vi "Fetch Class Documentation.vi"(8 "error in":errorcluster {"code" format="Error %.0f"}, 10 "Parser Settings":T1, 11 "Class in":refnum<vi>) -> (0 "error out":errorcluster {"code" format="Error %.0f"}, 3 "Class Documentation Out":refnum<class "Class Documentation.lvclass">)   [LabVIEW 2023, in "VIDoc Parsing.lvlib" / "Class Documentation.lvclass"]
doc: "Takes a Class Reference in and parses out all Class Documentation information needed for document generation."
uses:
  Class Documentation.lvclass
  Settings/Parser Settings/Parser Settings Cluster.ctl
  Settings/Parser Settings/Draw Controls Cluster.ctl
  Settings/Parser Settings/Draw Option Enum.ctl
  Class Documentation.lvclass/Class Documentation.ctl
  c4881257-149c-4e35-87db-cabb12afb1ac.vi
  VIDoc Parsing.lvlib
  Settings/Parser Settings/Parser Settings.lvclass
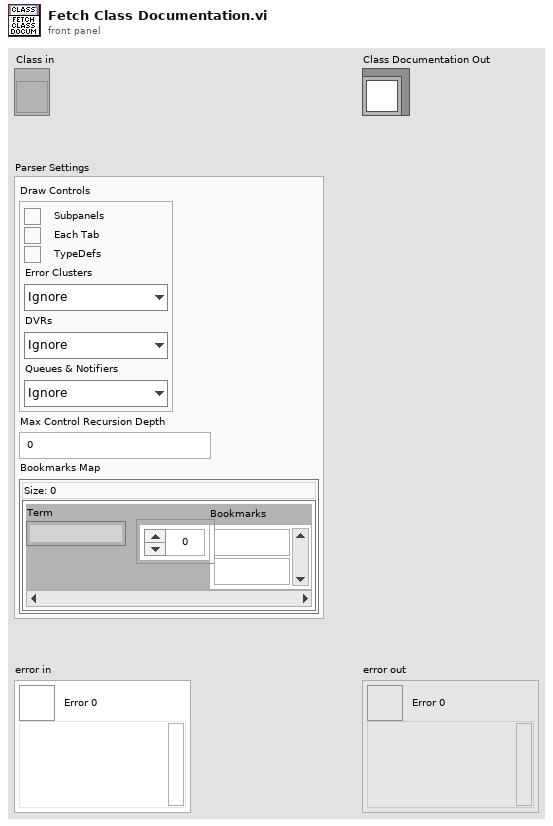
[diagram p1: front panel]
types:
  T1 = typedef "VIDoc Parsing.lvlib/Parser Settings.lvclass/Parser Settings Cluster.ctl" = cluster{"Draw Controls":T2, "Max Control Recursion Depth":i32, "Bookmarks Map":map{string, string[]}}
  T2 = typedef "VIDoc Parsing.lvlib/Parser Settings.lvclass/Draw Controls Cluster.ctl" = cluster{"Subpanels":bool, "Tabs":bool, "TypeDefs":bool, "Error Clusters":T3, "DVRs":T3, "Queues & Notifiers":T3}
  T3 = typedef "VIDoc Parsing.lvlib/Parser Settings.lvclass/Draw Option Enum.ctl" = enum16{"Ignore", "Draw", "Draw + Contents"}
  T4 = typedef "NI.Parent Library Information.ctl" = cluster{"qualified name":string, "localized name":string, "path":path, "parent library kind":T5}
  T5 = typedef "NI.Parent Library Kind.ctl" = enum32{"unknown", "class", "interface"}
  T6 = typedef "VIDoc Parsing.lvlib/Base Class Info Cluster.ctl" = cluster{"Name":string, "Icon":T7, "Version":cluster{"Major":u16, "Minor":u16, "Fix":u16, "Build":u16}, "Description":string, "Friends":string[], "ChildRefsRestricted":bool, "TransferMustOverrides":bool, "Path":path, "Qualified Name":string, "Class Scope":enum32{"invalid scope", "public", "private", "protected", "community"}}
  T7 = typedef "imagedata.ctl" = cluster{"image type":i32, "image depth":i32, "image":u8[], "mask":u8[], "colors":u32[], "Rectangle":cluster{"left":i16, "top":i16, "right":i16, "bottom":i16}}
  T8 = typedef "VIDoc Parsing.lvlib/Method Spec Cluster.ctl" = cluster{"VI Type Ext":T9, "Name":string, "Path":path, "Get Conpane Image":T7, "Description":string, "Get Library Access Scope":enum32{"invalid scope", "public", "private", "protected", "community"}, "Dispatch":T10, "ContainsCompiledCode":bool, "Exec.IsReentrant":bool, "Exec.ReentrancyType":enum16{"Share clones between instances", "Preallocate clone for each instance"}, "ExecInlining":bool, "ExecInlineIfPossible":bool, "Auto Err Handling":bool, "CodeComplexity":sgl, "Bookmark Tags":string[], "Control VI Type":enum32{"not a control VI", "control", "typedef", "strict typedef"}, "Controls":T11[], "VI Type":enum32{"invalid VI type", "Standard VI", "Control VI", "Global VI", "Polymorphic VI", "Configuration VI", "SubSystem", "Facade VI", "Method VI", "Statechart Diagram VI"}, "Minimum Size":T13, "Front Panel Window:Title":string, "Front Panel Window:Behavior":enum32{"Invalid", "Default", "Floating", "Floating/Auto-Hide", "Modal"}, "Front Panel Window:Closeable":bool, "Must Override":bool, "Must Use Parent Implementation":bool, "VI Icon":T7, "Front Panel":T7, "History:Revision Number":u32, "Metrics:Total Data Size":u32, "Execution:Allow Debugging":bool, "Execution:Preferred Exec System":enum32{"invalid execution system", "user interface", "standard", "instrument i/o", "data acquisition", "other 1", "other 2", "same as caller"}, "Execution:Priority":enum32{"invalid priority", "background priority", "normal priority", "above normal priority", "high priority", "time critical priority", "subroutine"}, "BM Tag Text":string[], "Block Diagram":T7, "Structure Tree":T14[]}
  T9 = typedef "VIDoc Parsing.lvlib/VI Type Extended Enum.ctl" = enum16{"Unknown", "Class Method", "Class Accessor Get", "Class Accessor Set", "Class Control", "Library Method", "Library Control", "VI", "Control"}
  T10 = typedef "VIDoc Parsing.lvlib/Class Dispatch Type Enum.ctl" = enum16{"None", "Static", "Dynamic"}
  T11 = typedef "VIDoc Parsing.lvlib/Controls Info Cluster.ctl" = cluster{"Name":string, "Description":string, "Data Type":string, "Tip Strip":string, "UID":i32, "Image Data":T7, "ToggleKeyBind":T12, "Raw Label":string, "Raw Caption":string}
  T12 = typedef "LVKeyTypeDef.ctl" = cluster{"Focus":bool, "Control":bool, "Shift":bool, "Key":string}
  T13 = typedef "LVPointTypeDef.ctl" = cluster{"Horizontal":i16, "Vertical":i16}
  T14 = typedef "VIDoc Parsing.lvlib/Structure Reporter.lvlib/Tree Cluster.ctl" = cluster{"Object Class Name":string, "Labels":string[], "Child Tag":string, "Item Indent":i32, "Child Only?":bool, "Glyph Index":i32}
  T15 = typedef "VIDoc Parsing.lvlib/Base Library Info Cluster.ctl" = cluster{"Name":string, "Icon":T7, "Version":cluster{"Major":u16, "Minor":u16, "Fix":u16, "Build":u16}, "Description":string, "Path":path, "Friends":string[], "Library Scope":enum32{"invalid scope", "public", "private", "protected", "community"}, "Qualified Name":string}
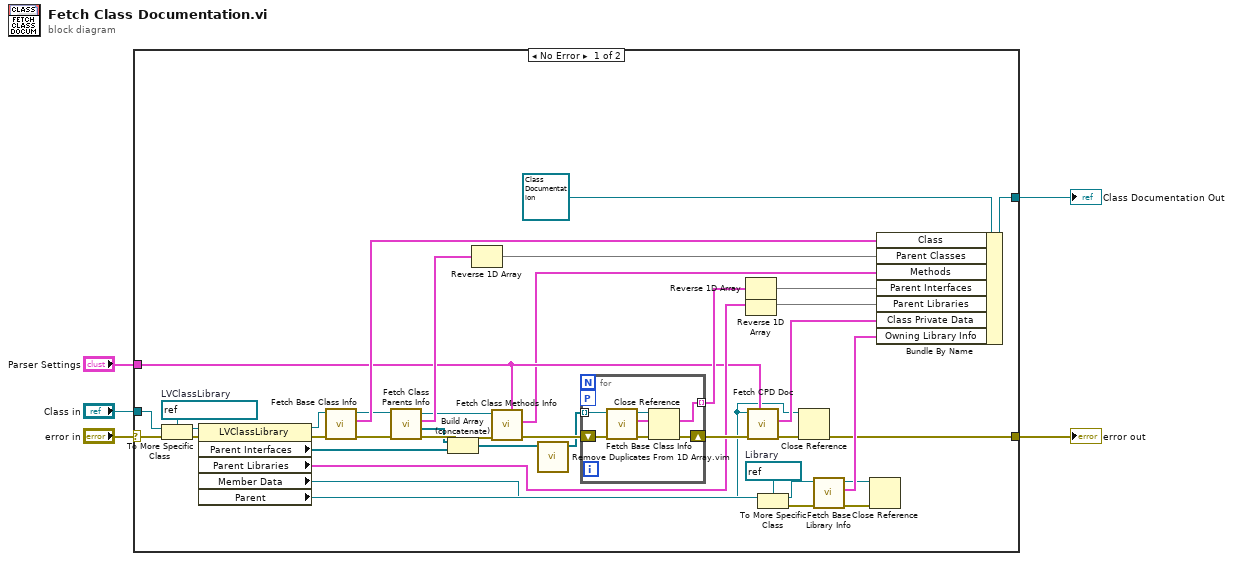
[diagram p0: block diagram]
diagram:
  n1 = case shown="No Error" "error in" {
    selector: "error in" -> [w44 w51]
    tunnel: [w9 w51] -> w4
    tunnel: "Class in" -> [w34 _]
    tunnel: [w32 _] -> w2
    tunnel: "Parser Settings" -> [w15 _]
    frame No Error {
      w13 = refnum<vi> refnum  # Library
      w35 = refnum<vi> refnum  # LVClassLibrary
      n2 = To More Specific Class(target class=w35, reference=w34, error in=w44) -> (specific class reference=w28:refnum<vi>, error out=w43:errorcluster)
      n3 = property class="LVClassLibrary"(reference=w28, error in=w43) -> (reference out=w27:refnum<vi>, error out=w41:errorcluster, "Parent Interfaces"=w25:refnum<vi>[], "Parent Libraries"=w19:T4[], "Member Data"=w8:refnum<vi>, "Parent"=w12:refnum<vi>)
      n4 = call "Fetch Base Class Info.vi"("error in (no error)"=w41, "LVClassLibrary in"=w27) -> ("error out"=w42:errorcluster, "Base Class Info"=w31:T6, "LVClassLibrary out"=w30:refnum<vi>)  [unwired: 7 in]
      n5 = call "Fetch Class Parents Info.vi"("error in (no error)"=w42, "LVClassLibrary in"=w30) -> ("error out"=w39:errorcluster, "Parent Interfaces"=w26:refnum<vi>[], "Parent Class Info"=w29:T6[], "LVClassLibrary out"=w16:refnum<vi>)  [unwired: 6 in]
      n6 = Build Array (concatenate)(w26, w25) -> (w24:refnum<vi>[])
      n7 = Reverse 1D Array(array=w29) -> (reversed array=w21:T6[])
      n8 = call "Fetch Class Methods Info.vi"("Parser Settings"=w15, "Error in"=w39, "LVClassLibrary"=w16) -> ("Error out"=w38:errorcluster, "Methods"=w14:T8[])  [unwired: 7 in]
      n9 = call "Remove Duplicates From 1D Array.vim"("array"=w24) -> ("array with duplicates removed"=w23:refnum<vi>[])  [unwired: 10 in]
      n10 = for {
        tunnel: [w47] -> w22 mode=indexing
        tunnel: w23 -> [w48] mode=indexing
        shift-right: [w46] -> w40
        shift-left: w38 -> [w50]
        workers-P: _ -> [_]
        n11 = call "Fetch Base Class Info.vi"("error in (no error)"=w50, "LVClassLibrary in"=w48) -> ("error out"=w49:errorcluster, "Base Class Info"=w47:T6, "LVClassLibrary out"=w45:refnum<vi>)  [unwired: 7 in]
        n12 = Close Reference(reference=w45, error in (no error)=w49) -> (error out=w46:errorcluster)
      }
      n13 = Reverse 1D Array(array=w22) -> (reversed array=w20:T6[])
      n14 = Reverse 1D Array(array=w19) -> (reversed array=w18:T4[])
      n15 = call "Fetch CPD Doc.vi"("Parser Settings"=w15, "error in"=w40, "VI in"=w8) -> ("error out"=w37:errorcluster, "Class Private Data"=w17:T11[])  [unwired: 7 in]
      n16 = To More Specific Class(target class=w13, reference=w12) -> (specific class reference=w11:refnum<vi>, error out=w36:errorcluster)  [unwired: 1 in]
      n17 = Close Reference(reference=w8, error in (no error)=w37) -> (error out=w9:errorcluster)
      n18 = call "Fetch Base Library Info.vi"("Error in"=w36, "Library in"=w11) -> ("Error out"=w6:errorcluster, "Base Library Info"=w10:T15, "Library out"=w7:refnum<vi>)  [unwired: 7 in]
      n19 = Close Reference(reference=w7, error in (no error)=w6) -> ()  [unwired: 1 out]
      n20 = Bundle By Name(cluster=refnum<class "Class Documentation.lvclass"> refnum ("Class Documentation out"), "Class"=w31, "Parent Classes"=w21, "Methods"=w14, "Parent Interfaces"=w20, "Parent Libraries"=w18, "Class Private Data"=w17, "Owning Library Info"=w10) -> (w32:refnum<class "Class Documentation.lvclass">)
    }
    frame Error {
    }
  }
  "error out" <- w4
  "Class Documentation Out" <- w2
